vi "Auto_Routine_Cube_Backup_Cube.vi"(8 "error in (no error)":errorcluster) -> (0 "error out":errorcluster)   [LabVIEW 2020]
uses:
  Arm/ArmPositionPreset.ctl
  Arm/ArmGamePiecePreset.ctl
  <vilib>/Rock Robotics/WPI/DriverStation/WPI_DriverStationAllianceInfo.ctl
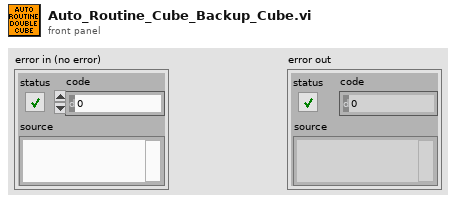
[diagram p1: front panel]
types:
  T1 = typedef "WPI_DriverStationAllianceInfo.ctl" = enum16{"Red", "Blue", "Invalid"}
  T2 = typedef "ArmGamePiecePreset.ctl" = enum16{"Cube", "Cone"}
  T3 = typedef "ArmPositionPreset.ctl" = enum16{"Upper", "Lower", "Middle", "Home", "Shelf", "Floor", "HalfFloor", "HalfHome"}
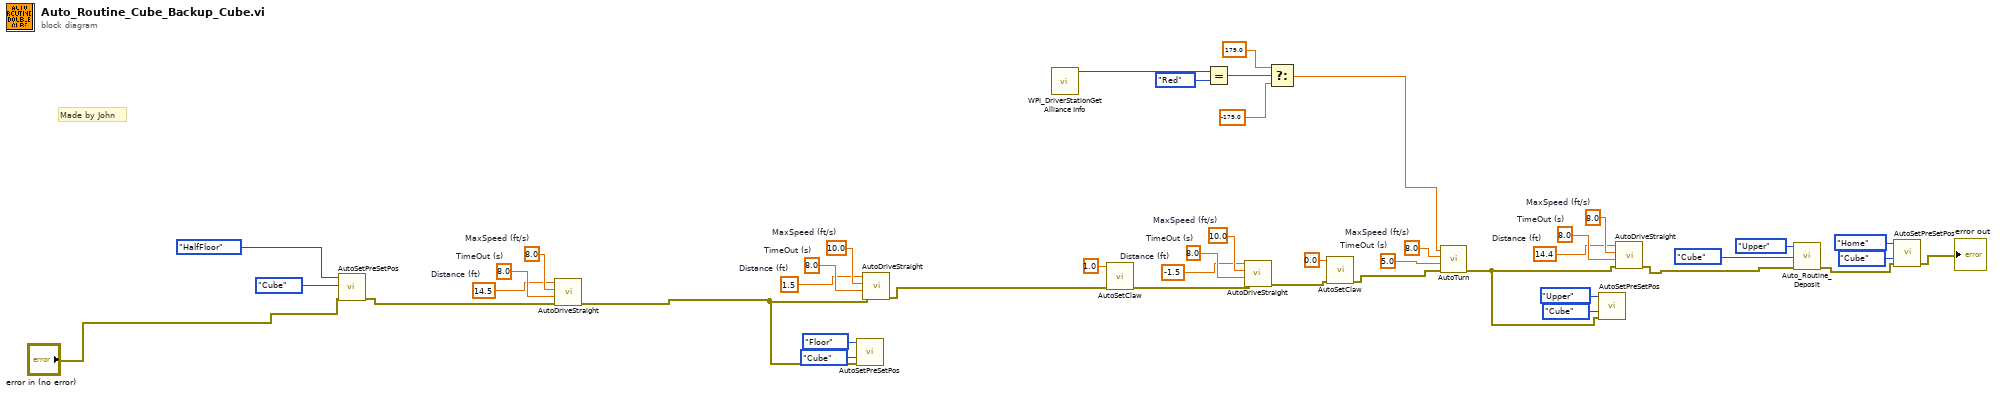
[diagram p0: block diagram]
diagram:
  w10 = 8.0  # TimeOut (s)
  w11 = 8.0  # MaxSpeed (ft/s)
  w9 = 14.4  # Distance (ft)
  w25 = 5.0  # TimeOut (s)
  w26 = 8.0  # MaxSpeed (ft/s)
  w30 = 8.0  # TimeOut (s)
  w31 = 10.0  # MaxSpeed (ft/s)
  w29 = -1.5  # Distance (ft)
  w33 = 8.0  # TimeOut (s)
  w34 = 10.0  # MaxSpeed (ft/s)
  w32 = 1.5  # Distance (ft)
  w42 = 8.0  # TimeOut (s)
  w43 = 8.0  # MaxSpeed (ft/s)
  w41 = 14.5  # Distance (ft)
  # "Made by John"
  n1 = call "AutoSetPreSetPos.vi"("error in (no error)"="error in (no error)", "Game Piece"=ArmGamePiecePreset."Cube", "Position"=ArmPositionPreset."HalfFloor") -> ("error out"=w12:errorcluster)  [unwired: 8 in]
  n2 = call "AutoDriveStraight.vi"("error in (no error)"=w12, "TimeOut (s)"=w42, "MaxSpeed (ft/s)"=w43, "Dist (ft)"=w41) -> ("error out"=w14:errorcluster)  [unwired: 7 in]
  n3 = call "AutoSetPreSetPos.vi"("error in (no error)"=w14, "Game Piece"=ArmGamePiecePreset."Cube", "Position"=ArmPositionPreset."Floor") -> ()  [unwired: 8 in, 1 out]
  n4 = call "AutoDriveStraight.vi"("error in (no error)"=w14, "TimeOut (s)"=w33, "MaxSpeed (ft/s)"=w34, "Dist (ft)"=w32) -> ("error out"=w15:errorcluster)  [unwired: 7 in]
  n5 = call <vilib>:"WPI_DriverStationGet Alliance Info.vi"() -> ("Alliance"=w6:T1)  [unwired: 6 in, 5 out]
  n6 = call "AutoSetClaw.vi"("error in (no error)"=w15, "ClawDemand"=1.0) -> ("error out"=w28:errorcluster)  [unwired: 9 in]
  n7 = Equal?(x=w6, y=WPI_DriverStationAllianceInfo."Red") -> (x = y?=w4:bool)
  n8 = call "AutoDriveStraight.vi"("error in (no error)"=w28, "TimeOut (s)"=w30, "MaxSpeed (ft/s)"=w31, "Dist (ft)"=w29) -> ("error out"=w27:errorcluster)  [unwired: 7 in]
  n9 = Select(t=179.0, s=w4, f=-179.0 ("degrees")) -> (s? t:f=w1:dbl)
  n10 = call "AutoSetClaw.vi"("error in (no error)"=w27, "ClawDemand"=0.0) -> ("error out"=w16:errorcluster)  [unwired: 9 in]
  n11 = call "AutoTurn.vi"("error in (no error)"=w16, "TimeOut (s)"=w25, "MaxSpeed (ft/s)"=w26, "degrees"=w1) -> ("error out"=w7:errorcluster)  [unwired: 7 in]
  n12 = call "AutoSetPreSetPos.vi"("error in (no error)"=w7, "Game Piece"=ArmGamePiecePreset."Cube", "Position"=ArmPositionPreset."Upper") -> ()  [unwired: 8 in, 1 out]
  n13 = call "AutoDriveStraight.vi"("error in (no error)"=w7, "TimeOut (s)"=w10, "MaxSpeed (ft/s)"=w11, "Dist (ft)"=w9) -> ("error out"=w8:errorcluster)  [unwired: 7 in]
  n14 = call "Auto_Routine_Deposit.vi"("error in (no error)"=w8, "Game Piece"=ArmGamePiecePreset."Cube", "Position"=ArmPositionPreset."Upper") -> ("error out"=w20:errorcluster)  [unwired: 8 in]
  n15 = call "AutoSetPreSetPos.vi"("error in (no error)"=w20, "Game Piece"=ArmGamePiecePreset."Cube", "Position"=ArmPositionPreset."Home") -> ("error out"=→"error out":errorcluster)  [unwired: 8 in]
